vi "subPrepareComplexPlot.vi"(11 "Array in":cdb[][](array[numeric])) -> (3 "Array out":dbl[][](array[numeric]))   [LabVIEW 2011]
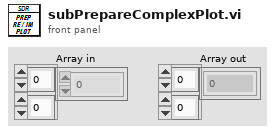
[diagram p1: front panel]
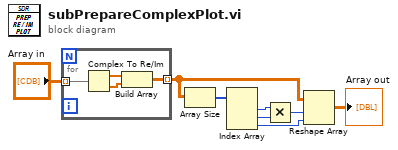
[diagram p0: block diagram]
diagram:
  n1 = for {
    tunnel: "Array in" -> [w12] mode=indexing
    tunnel: [w9] -> w1 mode=indexing
    n2 = Complex To Re/Im(x + iy=w12) -> (x=w11:dbl[], y=w10:dbl[])
    n3 = Build Array(w11, w10) -> (w9:dbl[][])
  }
  n4 = Array Size(array=w1) -> (size(s)=w7:i32[])
  n5 = Index Array(array=w7) -> (element #1=w5:i32, element #2=w4:i32, element #3=w3:i32)  [unwired: 3 in]
  n6 = Multiply(x=w5, y=w4) -> (x*y=w2:i32)
  n7 = Reshape Array(w1, w2, w3) -> (→"Array out":dbl[][])
